vi "Serial Comms - Initialise object.vi"(8 "error in (no error)":errorcluster, 9 "Connection Name":string, 10 "Serial Settings":T1={"VISA resource name "="", "baud rate"=9600, "data bits"=8, "parity"=enum."None", "stop bits"=10, "flow control"=0, "Timeout"=0, "termination char\n(0xA = '\\n' = LF) "=10, "Enable Termination Character"=FALSE} {"flow control" items=["None"=0, "XON/XOFF"=1, "RTS/CTS"=2, "DTR/DSR"=4]; "stop bits" items=["1.0"=10, "1.5"=15, "2.0"=20]; "data bits" min=5 max=8 step=1; "baud rate" items=["75"=75, "110"=110, "134"=134, "150"=150, "300"=300, "600"=600, "1200"=1200, "1800"=1800, "2400"=2400, "4800"=4800, "7200"=7200, "9600"=9600, "14400"=14400, "19200"=19200, "28800"=28800, "38400"=38400, "56000"=56000, "57600"=57600, "115200"=115200, "128000"=128000, "230400"=230400]}, 11 "Serial Comms in":refnum<class "Serial Comms.lvclass">) -> (0 "error out":errorcluster, 3 "Serial Comms out":refnum<class "Serial Comms.lvclass">)   [LabVIEW 2020, in "Generic_Comms.lvlib" / "Serial Comms.lvclass"]
uses:
  Serial Comms.lvclass
  Serial - Settings.ctl
  Serial Comms.lvclass/Serial Comms.ctl
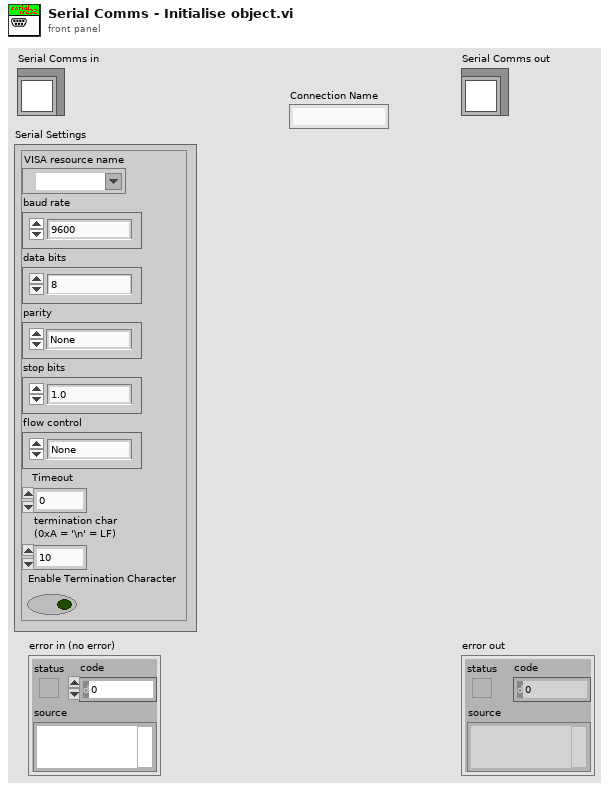
[diagram p1: front panel]
types:
  T1 = typedef "Serial - Settings.ctl" = cluster{"VISA resource name ":refnum<visa-resource-name>, "baud rate":u32, "data bits":u16, "parity":enum16{"None", "Odd", "Even", "Mark", "Space"}, "stop bits":u16, "flow control":u16, "Timeout":u32, "termination char\n(0xA = '\\n' = LF) ":u8, "Enable Termination Character":bool}
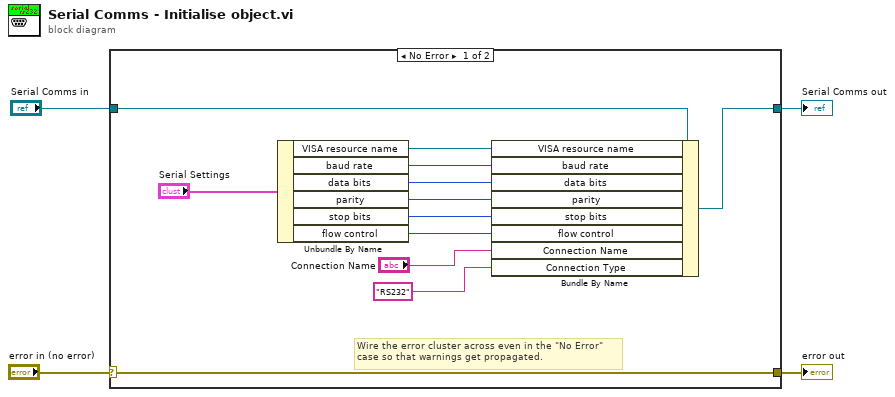
[diagram p0: block diagram]
diagram:
  n1 = case shown="No Error" "error in (no error)" {
    selector: "error in (no error)" -> [w16 w18]
    tunnel: [w16 w18] -> w3
    tunnel: [w15 w17] -> w1
    tunnel: "Serial Comms in" -> [w6 w17]
    frame No Error {
      # "Wire the error cluster across even in the \"No Error\"\ncase so that warnings get propagated."
      n2 = Unbundle By Name("Serial Settings") -> ("VISA resource name"=w13:refnum<visa-resource-name>, "baud rate"=w12:u32, "data bits"=w11:u16, "parity"=w10:enum16{"None", "Odd", "Even", "Mark", "Space"}, "stop bits"=w9:u16, "flow control"=w8:u16)
      n3 = Bundle By Name(cluster=w6, "VISA resource name"=w13, "baud rate"=w12, "data bits"=w11, "parity"=w10, "stop bits"=w9, "flow control"=w8, "Connection Name"="Connection Name", "Connection Type"="RS232") -> (w15:refnum<class "Serial Comms.lvclass">)
    }
    frame Error {
    }
  }
  "error out" <- w3
  "Serial Comms out" <- w1
